vi "M06 Power Plant.vi"(11 "EV3 in":T1) -> (1 "Angle out":sgl, 3 "EV3 out":T1)   [LabVIEW 2016]
uses:
  <vilib>/NXT/Subs/LVHSConnector.ctl
  <vilib>/NXT/LegoClasses/BrickReference/BrickReference.lvclass
  <vilib>/NXT/Dual Mode Library/Waits/Wait_Num.vi
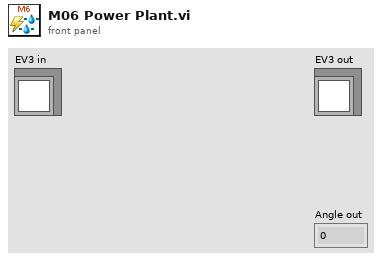
[diagram p1: front panel]
types:
  T1 = typedef "LVHSConnector.ctl" = refnum<class "BrickReference.lvclass">
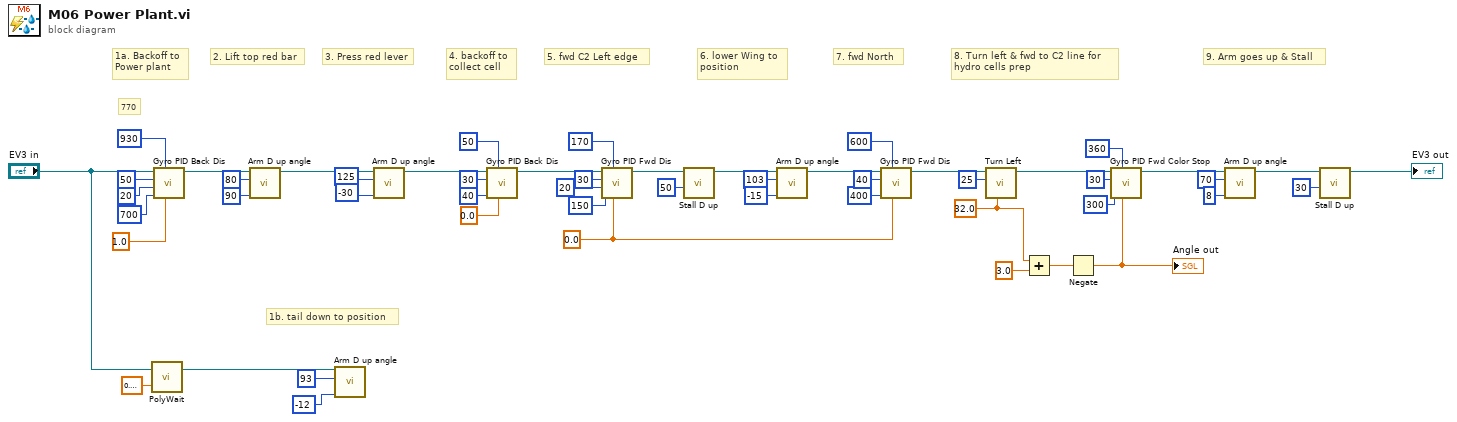
[diagram p0: block diagram]
diagram:
  w24 = sgl 0.0 ("Target angle")
  w14 = sgl 32.0 ("Turning angle")
  # "770"
  # "7. fwd North"
  # "4. backoff to\ncollect cell"
  # "6. lower Wing to\nposition"
  # "5. fwd C2 Left edge"
  # "9. Arm goes up & Stall"
  # "8. Turn left & fwd to C2 line for\nhydro cells prep"
  # "3. Press red lever"
  # "2. Lift top red bar"
  # "1b. tail down to position"
  # "1a. Backoff to\nPower plant"
  n1 = call-poly <vilib>:"PolyWait.vi"("Time (1 sec)"=sgl 0.7, "NXT/EV3"="EV3 in") -> ("NXT/EV3"=w2:T1)  [unwired: 2 in]
  n2 = call "Gyro PID Back Dis.vi"("Target angle"=sgl 1.0, "Threshold to stop"=930, "Threshold to slow"=700, "Min. speed"=20, "Max. speed"=50, "EV3 in"="EV3 in") -> ("EV3 out"=w36:T1)  [unwired: 5 in]
  n3 = call "Arm D up angle.vi"("Power"=i8 90, "Rotation"=80, "EV3 in"=w36) -> ("EV3 out"=w31:T1)  [unwired: 8 in]
  n4 = call "Arm D up angle.vi"("Power"=i8 -12, "Rotation"=93, "EV3 in"=w2) -> ()  [unwired: 8 in, 1 out]
  n5 = call "Arm D up angle.vi"("Power"=i8 -30, "Rotation"=125, "EV3 in"=w31) -> ("EV3 out"=w17:T1)  [unwired: 8 in]
  n6 = call "Gyro PID Back Dis.vi"("Target angle"=sgl 0.0, "Threshold to stop"=50, "Threshold to slow"=40, "Max. speed"=30, "EV3 in"=w17) -> ("EV3 out"=w16:T1)  [unwired: 6 in]
  n7 = call "Gyro PID Fwd Dis.vi"("Target angle"=w24, "Threshold to stop"=170 ("Threshold to Color"), "Threshold to slow"=150, "Min. speed"=20, "Max. speed"=30, "EV3 in"=w16) -> ("EV3 out"=w5:T1)  [unwired: 5 in]
  n8 = call "Stall D up.vi"("Power"=i8 50, "NXT/EV3"=w5) -> ("NXT/EV3"=w4:T1)  [unwired: 9 in]
  n9 = call "Arm D up angle.vi"("Power"=i8 -15, "Rotation"=103, "EV3 in"=w4) -> ("EV3 out"=w28:T1)  [unwired: 8 in]
  n10 = call "Gyro PID Fwd Dis.vi"("Target angle"=w24, "Threshold to stop"=600, "Threshold to slow"=400, "Max. speed"=40, "EV3 in"=w28) -> ("EV3 out"=w23:T1)  [unwired: 6 in]
  n11 = call "Turn Left.vi"("Turning angle"=w14, "Motor B (right)"=i8 25, "EV3 in"=w23) -> ("EV3 out"=w15:T1)  [unwired: 8 in]
  n12 = Add(x=w14, y=sgl 3.0) -> (x+y=w12:sgl)
  n13 = Negate(x=w12) -> (-x=w11:sgl)
  "Angle out" <- w11
  n14 = call "Gyro PID Fwd Color Stop.vi"("Target angle"=w11, "Threshold to Color"=360 ("Threshold to stop"), "Threshold to slow"=300, "Max. speed"=30, "EV3 in"=w15) -> ("EV3 out"=w10:T1)  [unwired: 6 in]
  n15 = call "Arm D up angle.vi"("Power"=i8 8, "Rotation"=70, "EV3 in"=w10) -> ("EV3 out"=w9:T1)  [unwired: 8 in]
  n16 = call "Stall D up.vi"("Power"=i8 30, "NXT/EV3"=w9) -> ("NXT/EV3"=→"EV3 out":T1)  [unwired: 9 in]
